vi "Read FPGA Ref.vi"(8 "error in (no error)":errorcluster, 11 "tCRD in":refnum<class "Aircraft OPCCRD.lvclass">) -> (0 "error out":errorcluster, 2 "FPGA Ref":T1, 3 "tCRD out":refnum<class "Aircraft OPCCRD.lvclass">)   [LabVIEW 2015, in "Aircraft OPCCRD.lvclass"]
uses:
  Aircraft OPCCRD.lvclass
  tFPGA Ref.ctl
  Aircraft OPCCRD.lvclass/Aircraft OPCCRD.ctl
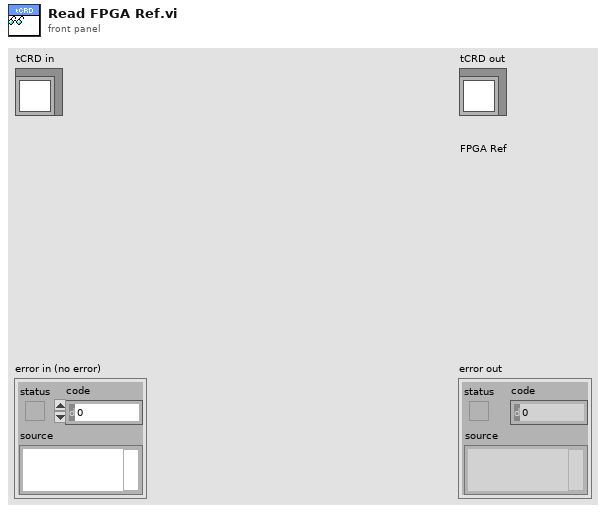
[diagram p1: front panel]
types:
  T1 = typedef "Aircraft OPCCRD.lvclass/tFPGA Ref.ctl" = refnum<k20>
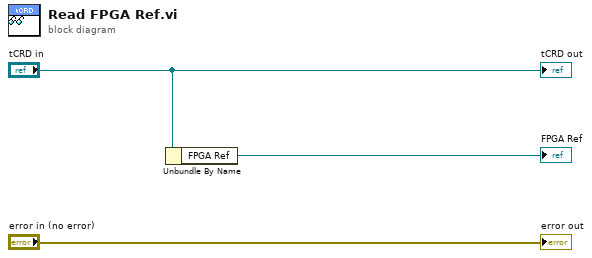
[diagram p0: block diagram]
diagram:
  n1 = Unbundle By Name("tCRD in") -> ("FPGA Ref"=→"FPGA Ref":T1)
  "error out" <- "error in (no error)"
  "tCRD out" <- "tCRD in"
